vi "Processing the actuator action.vi"(7 "error in (no error)":errorcluster, 8 "Actuator Name":string, 9 "Time to wait":i32=999, 10 "UTP IO Session in":T1) -> (0 "error out":errorcluster, 2 "Elapsed TimeToWait?":bool, 3 "UTP IO Session out":T1)   [LabVIEW 2023, in "Actuators.lvlib"]
doc: "Processing actutor action\nPeriod for reading is 10ms"
uses:
  Actuators.lvlib
  <vilib>/Noffz/UTP IO/UTP IO Library/Typedefs/Session Handle.ctl
  <vilib>/Noffz/UTP IO/UTP IO Library/UTP IO Pool Session.lvclass
  <vilib>/Noffz/UTP IO/UTP IO Library/methods/poly/plc/Write PLC Variable (Boolean).vi
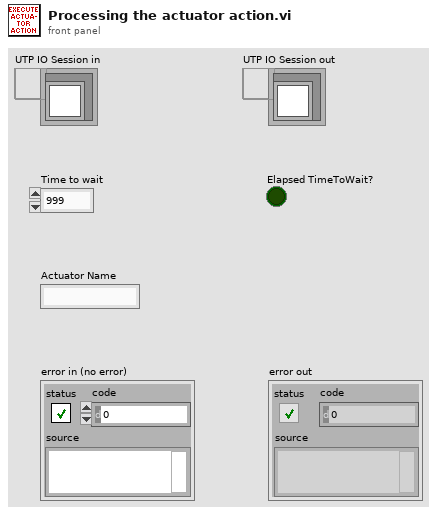
[diagram p1: front panel]
types:
  T1 = typedef "UTP IO Library.lvlib/UTP IO Pool Session.lvclass/Session Handle.ctl" = refnum<data-value>
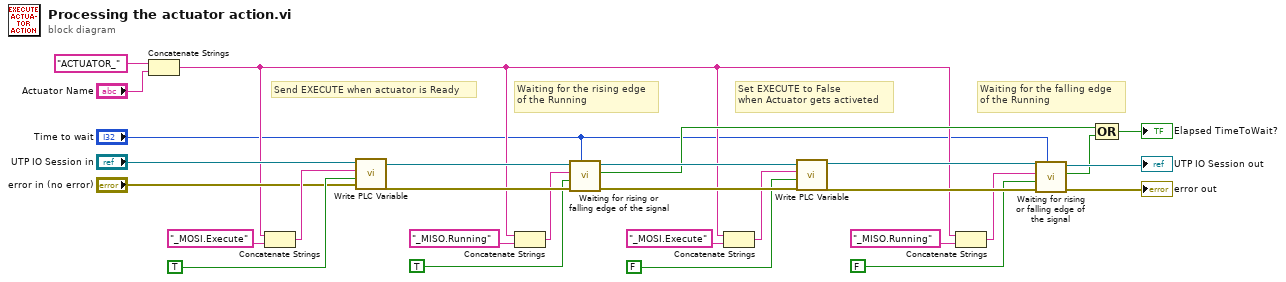
[diagram p0: block diagram]
diagram:
  # "Waiting for the falling edge\nof the Running"
  # "Set EXECUTE to False \nwhen Actuator gets activeted"
  # "Waiting for the rising edge\nof the Running"
  # "Send EXECUTE when actuator is Ready"
  n1 = Concatenate Strings("ACTUATOR_" ("string"), "Actuator Name") -> (w3:string)
  n2 = Concatenate Strings(w3, "_MOSI.Execute" ("string")) -> (w29:string)
  n3 = call-poly <vilib>:"Write PLC Variable.vi"("error in (no error)"="error in (no error)", "value"=TRUE, "variable name"=w29, "UTP IO Session in"="UTP IO Session in") -> ("error out"=w25:errorcluster, "UTP IO Session out"=w26:T1)  [unwired: 6 in]
  n4 = Concatenate Strings(w3, "_MISO.Running" ("string")) -> (w23:string)
  n5 = call "Waiting for rising or falling edge of the signal.vi"("Time to wait"="Time to wait", "error in"=w25, "Rising/Falling edge"=TRUE, "Variable name"=w23, "UTP IO Session in"=w26) -> ("error out"=w20:errorcluster, "ExpiredTimeToWait?"=w6:bool, "UTP IO Session out"=w21:T1)  [unwired: 4 in]
  n6 = Concatenate Strings(w3, "_MOSI.Execute" ("string")) -> (w18:string)
  n7 = call-poly <vilib>:"Write PLC Variable.vi"("error in (no error)"=w20, "value"=FALSE, "variable name"=w18, "UTP IO Session in"=w21) -> ("error out"=w15:errorcluster, "UTP IO Session out"=w16:T1)  [unwired: 6 in]
  n8 = Concatenate Strings(w3, "_MISO.Running" ("string")) -> (w13:string)
  n9 = call "Waiting for rising or falling edge of the signal.vi"("Time to wait"="Time to wait", "error in"=w15, "Rising/Falling edge"=FALSE, "Variable name"=w13, "UTP IO Session in"=w16) -> ("error out"=→"error out":errorcluster, "ExpiredTimeToWait?"=w7:bool, "UTP IO Session out"=→"UTP IO Session out":T1)  [unwired: 4 in]
  n10 = Compound Arithmetic op=OR(w6, w7) -> (→"Elapsed TimeToWait?":bool)
